vi "Sub_Report_Generation.vi"(8 "error in (no error)":errorcluster caption="에러 입력(에러 없음)", 11 "File Name":string) -> (0 "error out":errorcluster caption="에러 출력")   [LabVIEW 2015]
uses:
  <vilib>/addons/_office/excel.llb/Excel Easy Table (num).vi
  <vilib>/Utility/NIReport.llb/NI_report.lvclass
  <vilib>/addons/_office/NI_ReportGenerationToolkit.lvlib
  <vilib>/Utility/NIReport.llb/Excel/NI_Excel.lvclass
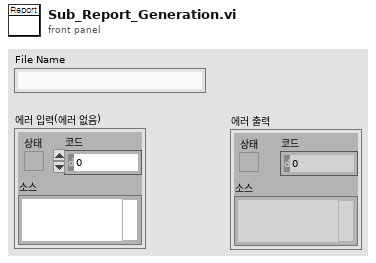
[diagram p1: front panel]
types:
  T1 = enum16{"Standard Report", "HTML", "Word", "Excel"}
  T2 = enum16{"maximized", "minimized", "normal", "no change"}
  T3 = cluster{"Load":dbl[], "LWA":dbl[], "LWB":dbl[], "LWC":dbl[], "RWA":dbl[], "RWB":dbl[], "RWC":dbl[], "Bat":u16[]}
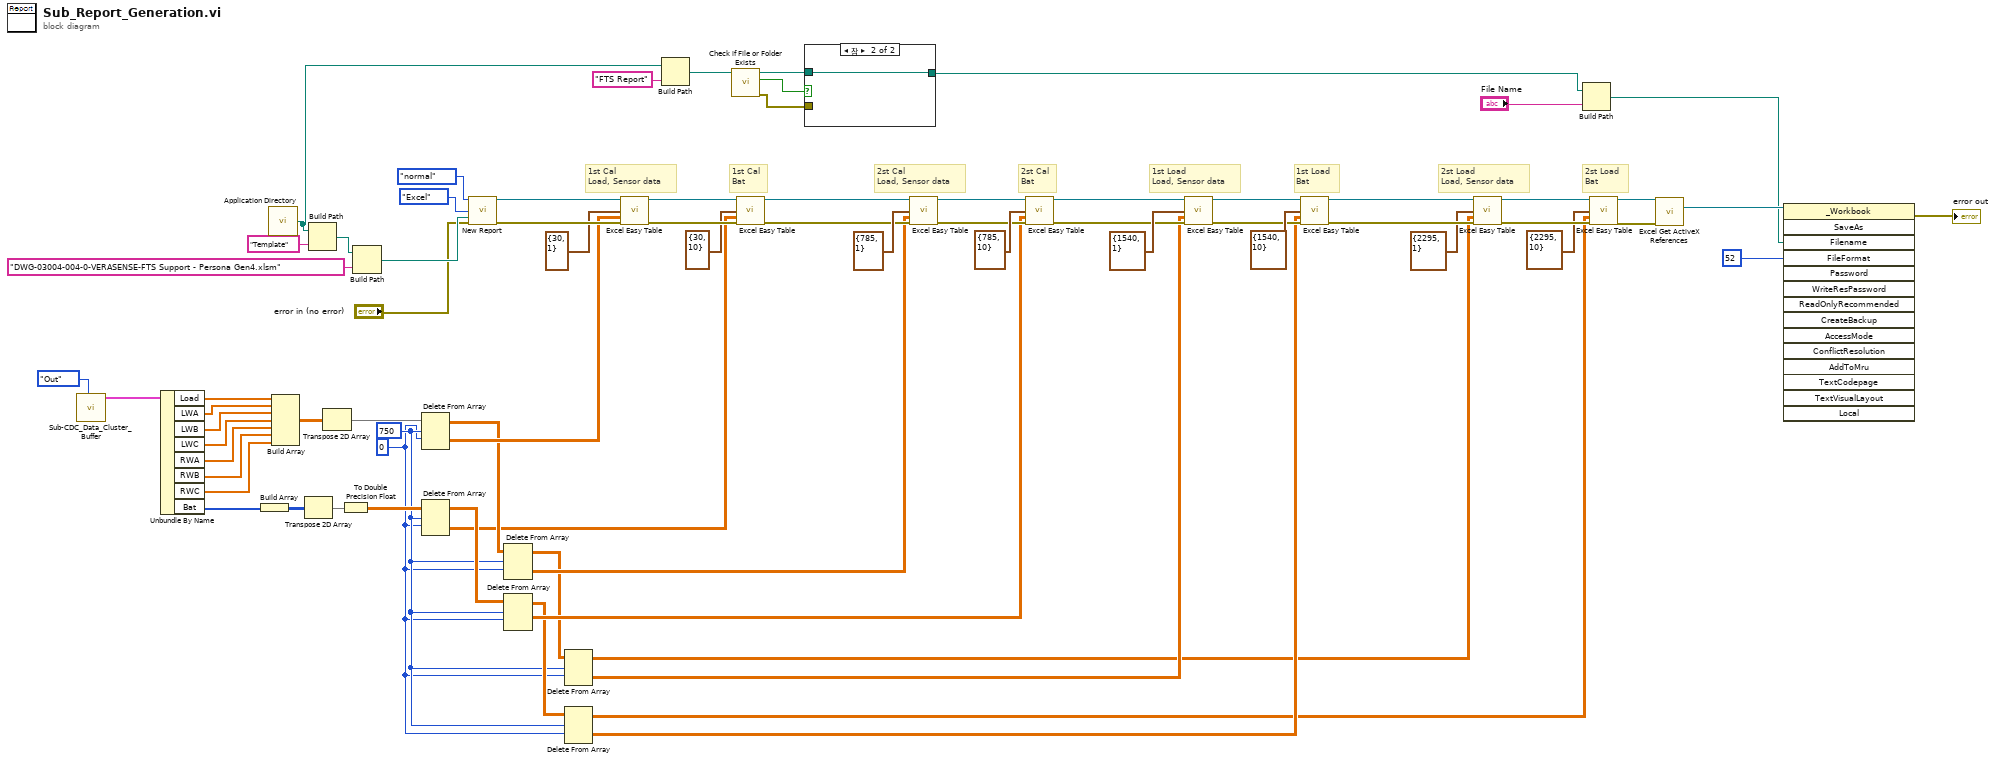
[diagram p0: block diagram]
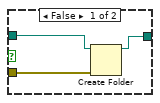
[diagram p2: hidden frame]
diagram:
  w20 = 0 ("인덱스 (행)")
  w21 = 750 ("길이")
  # "2st Load\nBat"
  # "2st Load\nLoad, Sensor data"
  # "1st Load\nBat"
  # "1st Load\nLoad, Sensor data"
  # "2st Cal\nBat"
  # "2st Cal\nLoad, Sensor data"
  # "1st Cal\nBat"
  # "1st Cal\nLoad, Sensor data"
  n1 = call "Sub-CDC_Data_Cluster_Buffer.vi"("Mode"=enum16{"Init", "Add", "Add Load", "Out"}."Out") -> ("Output CL"=w65:T3)  [unwired: 10 in]
  n2 = Unbundle By Name(w65) -> ("Load"=w64:dbl[], "LWA"=w63:dbl[], "LWB"=w62:dbl[], "LWC"=w61:dbl[], "RWA"=w60:dbl[], "RWB"=w59:dbl[], "RWC"=w58:dbl[], "Bat"=w39:u16[])
  n3 = Build Array(w39) -> (w50:u16[][])
  n4 = call <vilib>:"Application Directory.vi"() -> ("Application Directory"=w15:path)
  n5 = Build Array(w64, w63, w62, w61, w60, w59, w58) -> (w57:dbl[][])
  n6 = Transpose 2D Array(2D array=w50) -> (transposed array=w49:u16[][])
  n7 = Build Path(base path=w15, name or relative path="Template" ("이름 또는 상대 경로")) -> (appended path=w71:path)
  n8 = Transpose 2D Array(2D array=w57) -> (transposed array=w56:dbl[][])
  n9 = To Double Precision Float(number=w49) -> (double precision float=w38:dbl[][])
  n10 = Build Path(base path=w71, name or relative path="DWG-03004-004-0-VERASENSE-FTS Support - Persona Gen4.xlsm" ("이름 또는 상대 경로")) -> (appended path=w69:path)
  n11 = Delete From Array(array=w56, length=w21, index (row)=w20) -> (deleted portion=w55:dbl[][], array with subset deleted=w48:dbl[][])  [unwired: 1 in]
  n12 = Delete From Array(array=w38, length=w21, index (row)=w20) -> (deleted portion=w36:dbl[][], array with subset deleted=w47:dbl[][])  [unwired: 1 in]
  n13 = call <vilib>:"New Report.vi"("window state (normal)"=T2."normal", "report type"=T1."Excel", "template (empty)"=w69, "error in (no error)"="error in (no error)") -> ("report out"=w68:refnum<class "NI_report.lvclass">, "error out"=w67:errorcluster)  [unwired: 10 in]
  n14 = Delete From Array(array=w48, length=w21, index (row)=w20) -> (deleted portion=w40:dbl[][], array with subset deleted=w23:dbl[][])  [unwired: 1 in]
  n15 = Delete From Array(array=w47, length=w21, index (row)=w20) -> (deleted portion=w37:dbl[][], array with subset deleted=w22:dbl[][])  [unwired: 1 in]
  n16 = Delete From Array(array=w23, length=w21, index (row)=w20) -> (deleted portion=w19:dbl[][], array with subset deleted=w17:dbl[][])  [unwired: 1 in]
  n17 = Delete From Array(array=w22, length=w21, index (row)=w20) -> (deleted portion=w18:dbl[][], array with subset deleted=w16:dbl[][])  [unwired: 1 in]
  n18 = call-poly <vilib>:"Excel Easy Table.vi"("report in"=w68, "start (0, 0)"=cluster{"row":i32, "column":i32} {"row"=30, "column"=1}, "text data"=w55, "error in (no error)"=w67) -> ("report out"=w53:refnum<class "NI_report.lvclass">, "error out"=w52:errorcluster)  [unwired: 7 in, 3 out]
  n19 = Build Path(base path=w15, name or relative path="FTS Report" ("이름 또는 상대 경로")) -> (appended path=w10:path)
  n20 = call <vilib>:"Check if File or Folder Exists.vi"("path"=w10) -> ("error out"=w11:errorcluster, "file or folder exists?"=w13:bool, "dup path"=w12:path)  [unwired: 8 in]
  n21 = call-poly <vilib>:"Excel Easy Table.vi"("report in"=w53, "start (0, 0)"=cluster{"row":i32, "column":i32} {"row"=30, "column"=10}, "text data"=w36, "error in (no error)"=w52) -> ("report out"=w42:refnum<class "NI_report.lvclass">, "error out"=w41:errorcluster)  [unwired: 7 in, 3 out]
  n22 = case shown="참" w13 {
    tunnel: w12 -> [w77 w78]
    tunnel: w11 -> [w76 _]
    tunnel: [w75 w78] -> w9
    frame False {
      n23 = Create Folder(path (use dialog)=w77, error in=w76) -> (created path=w75:path)  [unwired: 1 in, 2 out]
    }
    frame True {
    }
  }
  n24 = call-poly <vilib>:"Excel Easy Table.vi"("report in"=w42, "start (0, 0)"=cluster{"row":i32, "column":i32} {"row"=785, "column"=1}, "text data"=w40, "error in (no error)"=w41) -> ("report out"=w44:refnum<class "NI_report.lvclass">, "error out"=w45:errorcluster)  [unwired: 7 in, 3 out]
  n25 = call-poly <vilib>:"Excel Easy Table.vi"("report in"=w44, "start (0, 0)"=cluster{"row":i32, "column":i32} {"row"=785, "column"=10}, "text data"=w37, "error in (no error)"=w45) -> ("report out"=w25:refnum<class "NI_report.lvclass">, "error out"=w24:errorcluster)  [unwired: 7 in, 3 out]
  n26 = call-poly <vilib>:"Excel Easy Table.vi"("report in"=w25, "start (0, 0)"=cluster{"row":i32, "column":i32} {"row"=1540, "column"=1}, "text data"=w19, "error in (no error)"=w24) -> ("report out"=w27:refnum<class "NI_report.lvclass">, "error out"=w28:errorcluster)  [unwired: 7 in, 3 out]
  n27 = call-poly <vilib>:"Excel Easy Table.vi"("report in"=w27, "start (0, 0)"=cluster{"row":i32, "column":i32} {"row"=1540, "column"=10}, "text data"=w18, "error in (no error)"=w28) -> ("report out"=w34:refnum<class "NI_report.lvclass">, "error out"=w35:errorcluster)  [unwired: 7 in, 3 out]
  n28 = call-poly <vilib>:"Excel Easy Table.vi"("report in"=w34, "start (0, 0)"=cluster{"row":i32, "column":i32} {"row"=2295, "column"=1}, "text data"=w17, "error in (no error)"=w35) -> ("report out"=w32:refnum<class "NI_report.lvclass">, "error out"=w31:errorcluster)  [unwired: 7 in, 3 out]
  n29 = Build Path(base path=w9, name or relative path="File Name") -> (appended path=w2:path)
  n30 = call-poly <vilib>:"Excel Easy Table.vi"("report in"=w32, "start (0, 0)"=cluster{"row":i32, "column":i32} {"row"=2295, "column"=10}, "text data"=w16, "error in (no error)"=w31) -> ("report out"=w5:refnum<class "NI_report.lvclass">, "error out"=w6:errorcluster)  [unwired: 7 in, 3 out]
  n31 = call <vilib>:"Excel Get ActiveX References.vi"("report in"=w5, "error in (no error)"=w6) -> ("Excel._Workbook"=w4:refnum<k7>)  [unwired: 7 in, 6 out]
  n32 = invoke on="인보크 노드" class="_Workbook" method="SaveAs"(reference=w4, "Filename"=w2, "FileFormat"=52) -> (error out=→"error out":errorcluster)  [unwired: 12 in, 14 out]
